vi "Building_Subtrack_Add_Part-1.vi"(4 "[IN] # Track with \nProblem Point":i32, 5 "[IN] Index of \nProblem Point":i32, 6 "error IN":errorcluster, 7 "[IN] Subtrack":T1, 8 "[IN] Last Point in Subtrack":i32, 9 "[IN] Still connected\ntracks in group":T2) -> (0 "error OUT":errorcluster, 1 "[OUT] Subtrack":T1, 2 "[OUT] Last point in subtrack":i32, 3 "[OUT] Index of Last\nStop Point in Track":i32)   [LabVIEW 2017]
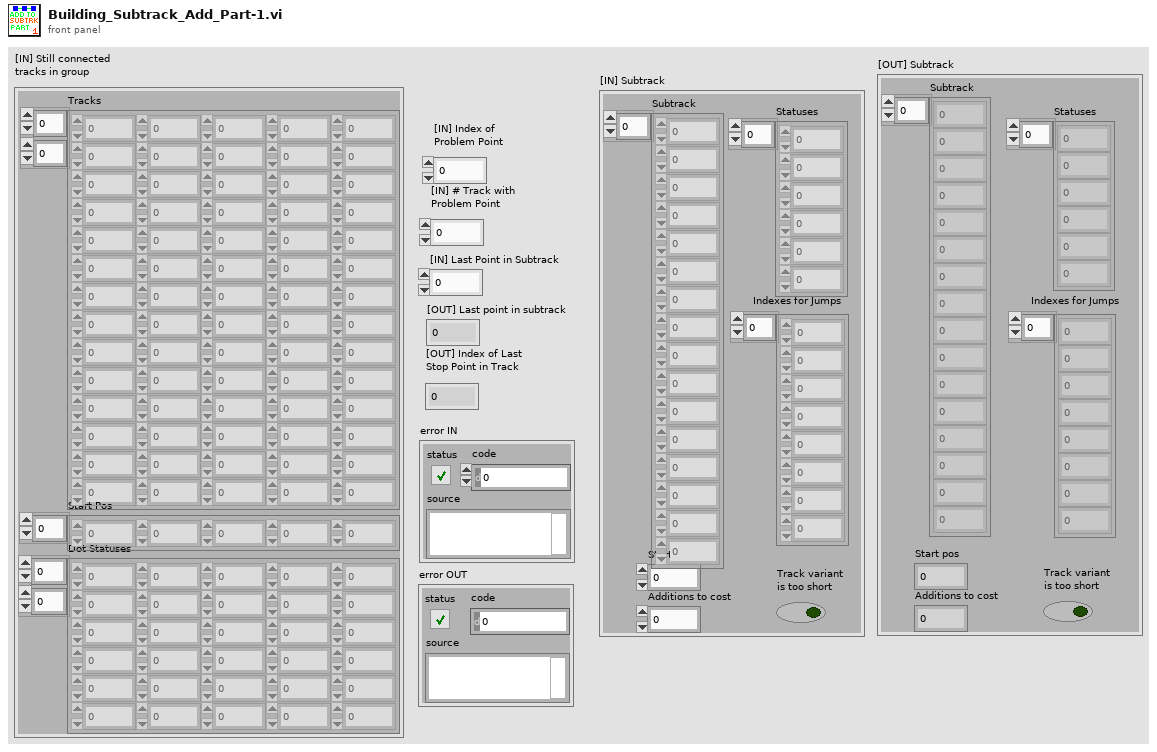
[diagram p1: front panel]
types:
  T1 = cluster{"Subtrack":dbl[], "Statuses":i16[], "Start pos":i32, "Additions to cost":i8, "Track variant \nis too short":bool, "Indexes for Jumps":i32[]}
  T2 = cluster{"Tracks":dbl[][], "Start Pos":i32[], "Dot Statuses":i16[][]}
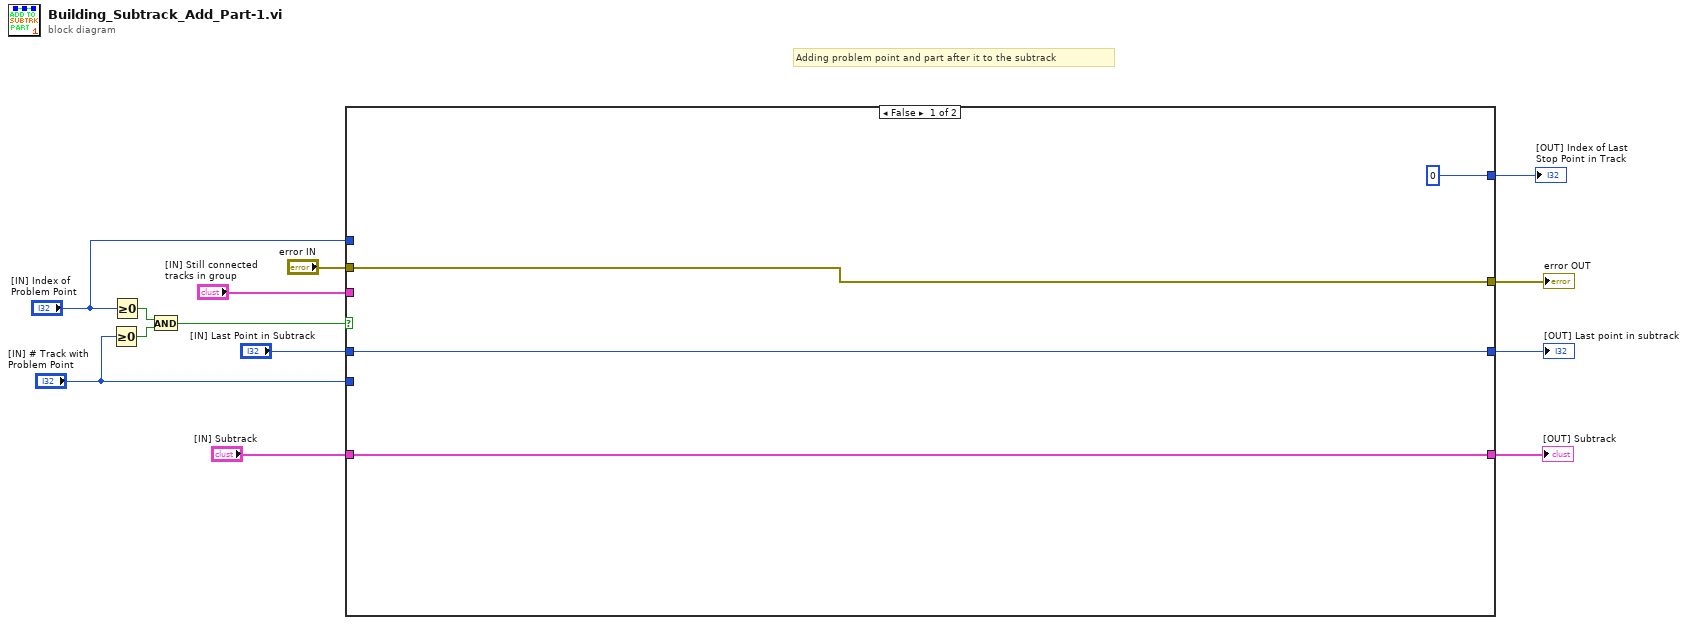
[diagram p0: block diagram]
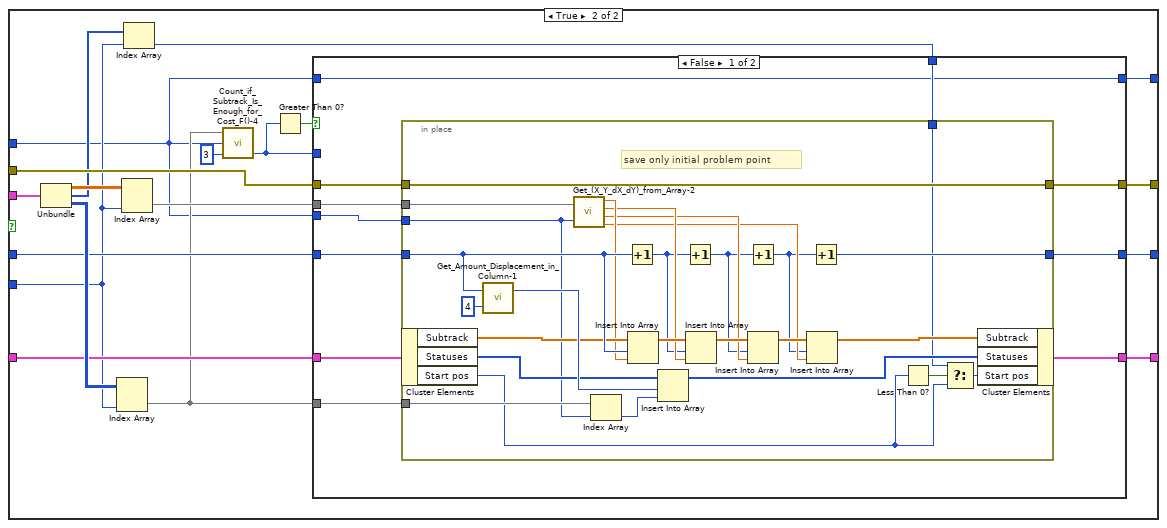
[diagram p2: hidden frame]
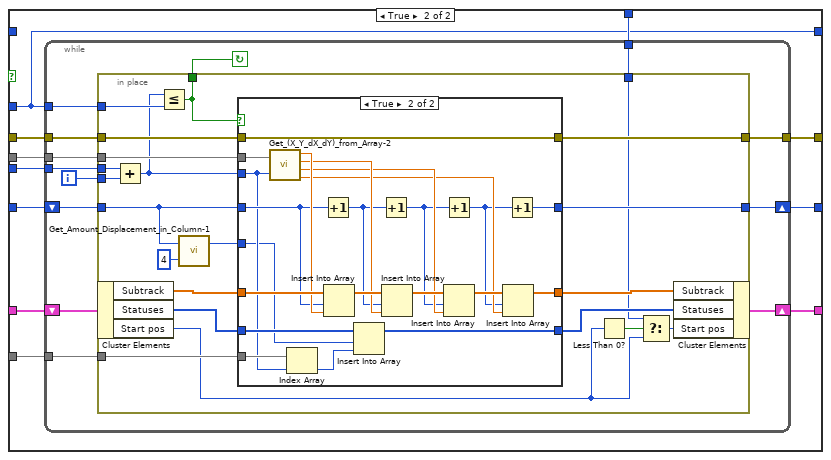
[diagram p3: hidden frame]
diagram:
  # "Adding problem point and part after it to the subtrack"
  n1 = Greater Or Equal To 0?(x="[IN] # Track with \nProblem Point") -> (x >= 0?=w7:bool)
  n2 = Greater Or Equal To 0?(x="[IN] Index of \nProblem Point") -> (x >= 0?=w8:bool)
  n3 = And(x=w8, y=w7) -> (x .and. y?=w6:bool)
  n4 = case shown="False" w6 {
    tunnel: "[IN] Still connected\ntracks in group" -> [_ w36]
    tunnel: [w15 w32] -> w12
    tunnel: [w17 w31] -> w11
    tunnel: "[IN] Subtrack" -> [w16 w30]
    tunnel: [w16 w29] -> w9
    tunnel: "[IN] # Track with \nProblem Point" -> [_ w23]
    tunnel: "error IN" -> [w17 w28]
    tunnel: "[IN] Last Point in Subtrack" -> [w15 w27]
    tunnel: "[IN] Index of \nProblem Point" -> [_ w18]
    tunnel: [0 ("[OUT] Index of Last \nPoint in Track") w19] -> w1
    frame False {
    }
    frame True {
      n5 = Unbundle(w36) -> ("Tracks"=w35:dbl[][], "Start Pos"=w24:i32[], "Dot Statuses"=w33:i16[][])
      n6 = Index Array(array=w33, index (col)=w23) -> (element=w26:i16[])  [unwired: 1 in]
      n7 = Index Array(array=w35, index (col)=w23) -> (element=w34:dbl[])  [unwired: 1 in]
      n8 = Index Array(array=w24, index=w23) -> (element=w22:i32)
      n9 = call "Count_if_Subtrack_Is_Enough_for_Cost_F()-4.vi"("[IN] Minimal Subtrack Length \n(Points without problems) for\nMaking Desicion"=3 ("[IN] Minimal Subtrack Length \n(Points without problems) for\nMaking Desicion"), "[IN] Index of Problem \nPoint Inside Track"=w18, "[IN] Dot Statuses in Track"=w26) -> ("[OUT] Index of Last \nPoint in Track"=w21:i32)  [unwired: 1 in, 1 out]
      n10 = Greater Than 0?(x=w21) -> (x > 0?=w20:bool)
      n11 = case shown="False" w20 {
        tunnel: w34 -> [w42 w85]
        tunnel: [w39 w84] -> w32
        tunnel: [w40 w83] -> w31
        tunnel: w30 -> [w47 w82]
        tunnel: [w38 w81] -> w29
        tunnel: w28 -> [w43 w80]
        tunnel: w27 -> [w45 w79]
        tunnel: w26 -> [w46 w78]
        tunnel: w21 -> [_ w75]
        tunnel: w22 -> [w41 w77]
        tunnel: w18 -> [w44 w76]
        tunnel: [w37 w75] -> w19
        tunnel: w18 -> [w37 _]
        frame False {
          n12 = in-place {
            in-place-border: w42 -> [w74]
            in-place-border: w46 -> [w73]
            in-place-border: w43 -> [w72]
            in-place-border: [w72] -> w40
            in-place-border: [w71] -> w39
            in-place-border: w45 -> [w69]
            in-place-border: w41 -> [w62]
            in-place-border: w44 -> [w59]
            # "save only initial problem point"
            n13 = in-place-cluster #1(w47) -> ("Subtrack"=w67:dbl[], "Statuses"=w66:i16[], "Start pos"=w60:i32)
            n14 = call "Get_Amount_Displacement_in_Column-1.vi"("multiplier"=4, "# Rows"=w69) -> ("Displ amount"=w68:i32)  [unwired: 1 out]
            n15 = call "Get_(X_Y_dX_dY)_from_Array-2.vi"("(X,Y,dX,dY)"=w74, "Index of Displacement"=w59) -> ("X"=w58:dbl, "Y"=w56:dbl, "dX"=w53:dbl, "dY"=w50:dbl)
            n16 = Index Array(array=w73, index=w59) -> (element=w49:i16)
            n17 = Increment(x=w69) -> (x+1=w54:i32)
            n18 = Insert Into Array(array=w67, index=w69, new element=w58) -> (w57:dbl[])
            n19 = Insert Into Array(array=w66, index=w68, new element=w49) -> (w64:i16[])
            n20 = Increment(x=w54) -> (x+1=w52:i32)
            n21 = Insert Into Array(array=w57, index=w54, new element=w56) -> (w55:dbl[])
            n22 = Increment(x=w52) -> (x+1=w48:i32)
            n23 = Insert Into Array(array=w55, index=w52, new element=w53) -> (w51:dbl[])
            n24 = Insert Into Array(array=w51, index=w48, new element=w50) -> (w65:dbl[])
            n25 = Increment(x=w48) -> (x+1=w71:i32)
            n26 = Less Than 0?(x=w60) -> (x < 0?=w63:bool)
            n27 = Select(t=w62, s=w63, f=w60) -> (s? t:f=w61:i32)
            n28 = in-place-cluster #1("Subtrack"=w65, "Statuses"=w64, "Start pos"=w61) -> (w38:T1)
          }
        }
        frame True {
          n29 = while {
            tunnel: w85 -> [w98]
            tunnel: w78 -> [w96]
            shift-right: [w89] -> w81
            shift-left: w82 -> [w90]
            tunnel: w80 -> [w94]
            tunnel: [w93] -> w83
            shift-right: [w92] -> w84
            shift-left: w79 -> [w91]
            tunnel: w75 -> [w86]
            tunnel: w77 -> [w88]
            tunnel: w76 -> [w87]
            i -> [w95]
            stop <- w97 continue-if-true
            n30 = in-place {
              in-place-border: w98 -> [w119]
              in-place-border: [w118] -> w97
              in-place-border: w96 -> [w117]
              in-place-border: w86 -> [w116]
              in-place-border: w95 -> [w100]
              in-place-border: w94 -> [w115]
              in-place-border: [w114] -> w93
              in-place-border: [w113] -> w92
              in-place-border: w91 -> [w111]
              in-place-border: w88 -> [w104]
              in-place-border: w87 -> [w101]
              n31 = in-place-cluster #2(w90) -> ("Subtrack"=w109:dbl[], "Statuses"=w108:i16[], "Start pos"=w102:i32)
              n32 = Add(x=w101, y=w100) -> (x+y=w99:i32)
              n33 = Less Or Equal?(x=w99, y=w116) -> (x <= y?=w118:bool)
              n34 = call "Get_Amount_Displacement_in_Column-1.vi"("multiplier"=4, "# Rows"=w111) -> ("Displ amount"=w110:i32)  [unwired: 1 out]
              n35 = case shown="True" w118 {
                tunnel: w119 -> [_ w145]
                tunnel: w109 -> [w122 w144]
                tunnel: w111 -> [w120 w142]
                tunnel: w99 -> [_ w131]
                tunnel: w108 -> [w123 w133]
                tunnel: w117 -> [_ w132]
                tunnel: [w122 w129] -> w107
                tunnel: [w123 w128] -> w106
                tunnel: w115 -> [w121 w127]
                tunnel: [w121 w127] -> w114
                tunnel: [w120 w124] -> w113
                tunnel: w110 -> [_ w126]
                frame False {
                }
                frame True {
                  n36 = call "Get_(X_Y_dX_dY)_from_Array-2.vi"("(X,Y,dX,dY)"=w145, "Index of Displacement"=w131) -> ("X"=w143:dbl, "Y"=w140:dbl, "dX"=w137:dbl, "dY"=w134:dbl)
                  n37 = Index Array(array=w132, index=w131) -> (element=w130:i16)
                  n38 = Increment(x=w142) -> (x+1=w138:i32)
                  n39 = Insert Into Array(array=w144, index=w142, new element=w143) -> (w141:dbl[])
                  n40 = Insert Into Array(array=w133, index=w126, new element=w130) -> (w128:i16[])
                  n41 = Increment(x=w138) -> (x+1=w136:i32)
                  n42 = Insert Into Array(array=w141, index=w138, new element=w140) -> (w139:dbl[])
                  n43 = Increment(x=w136) -> (x+1=w125:i32)
                  n44 = Insert Into Array(array=w139, index=w136, new element=w137) -> (w135:dbl[])
                  n45 = Insert Into Array(array=w135, index=w125, new element=w134) -> (w129:dbl[])
                  n46 = Increment(x=w125) -> (x+1=w124:i32)
                }
              }
              n47 = Less Than 0?(x=w102) -> (x < 0?=w105:bool)
              n48 = Select(t=w104, s=w105, f=w102) -> (s? t:f=w103:i32)
              n49 = in-place-cluster #2("Subtrack"=w107, "Statuses"=w106, "Start pos"=w103) -> (w89:T1)
            }
          }
        }
      }
    }
  }
  "[OUT] Last point in subtrack" <- w12
  "error OUT" <- w11
  "[OUT] Subtrack" <- w9
  "[OUT] Index of Last\nStop Point in Track" <- w1
